vi "Get HW type.vi"(7 "Comm":T1, 8 "error in (no error)":errorcluster) -> (0 "error out":errorcluster, 3 "hwDefaultSetting":T2)   [LabVIEW 2016]
uses:
  Controls/hwDefaultSetting.ctl
  Controls/hwSettings command.ctl
  <vilib>/Utility/config.llb/Read Key (String).vi
  <vilib>/Utility/config.llb/Read Key (U32).vi
  <vilib>/Utility/config.llb/NI_LVConfig.lvlib
panel:
  # "[hw]\nType=Simulation\nhwNumber=2\nhwName=MX840A-1,MX840A-2\nhwSN=0009E5009B32,0009E5009B33\nhwCHNumber=8,8"
  # "I:\\0. iAmleoCHO\\0.09 Projects_ZCJX\\2017\\3. 6Y11S_ZMS_液流台&热气台数据采集\\ZcDAQ\\E\\LabviewPrj\\曹队\\ZcDAQprj\\Builds\\Configuration\n\nI:\\0. iAmleoCHO\\0.09 Projects_ZCJX\\2017\\3. 6Y11S_ZMS_液流台&热气台数据采集\\ZcDAQ\\E\\LabviewPrj\\曹队\\ZcDAQprj\\Builds\\Configuration\\hwtype.ini"
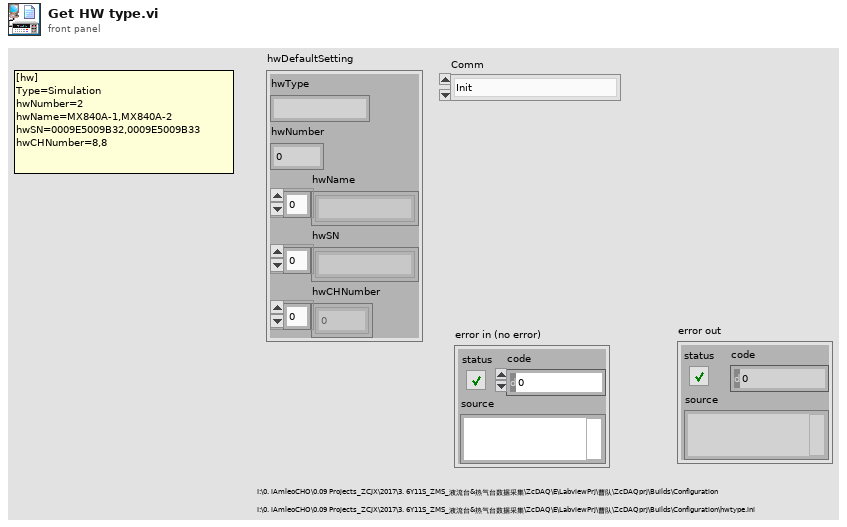
[diagram p1: front panel]
types:
  T1 = typedef "hwSettings command.ctl" = enum16{"Init", "Read", "Clear"}
  T2 = typedef "hwDefaultSetting.ctl" = cluster{"hwType":string, "hwNumber":u32, "hwName":string[], "hwSN":string[], "hwCHNumber":u32[]}
  T3 = cluster{"TREE PNG":path, "User Guide":path, "DefaultSave":path, "BuildPath":path, "Image":path, "Modules":path, "Configuration":path, "License":path, "SplitFiles":path, "System.ini":path}
  T4 = typedef "NI_LVConfig.lvlib/Config Data RefNum.ctl" = refnum<k1>
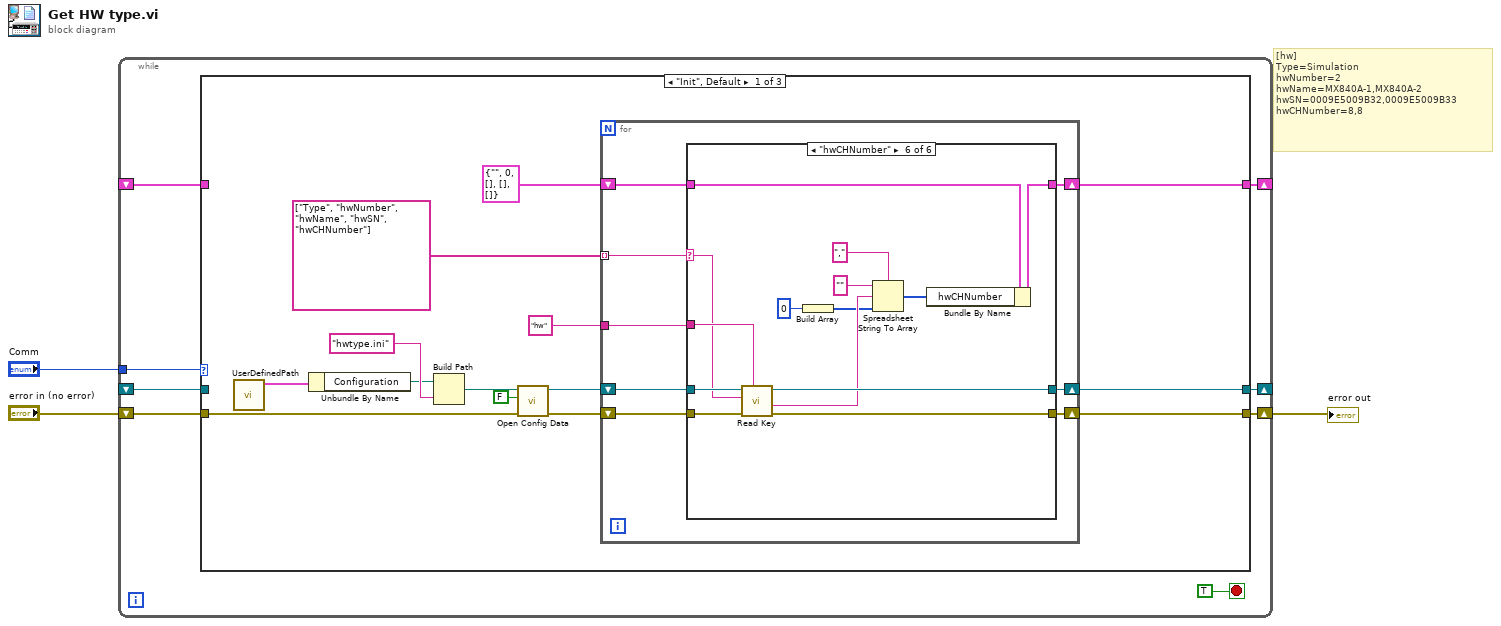
[diagram p0: block diagram]
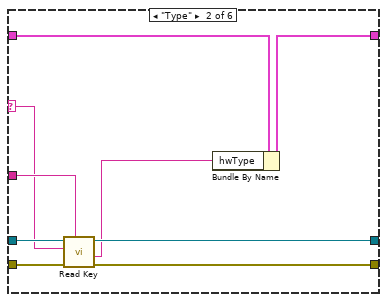
[diagram p3: hidden frame]
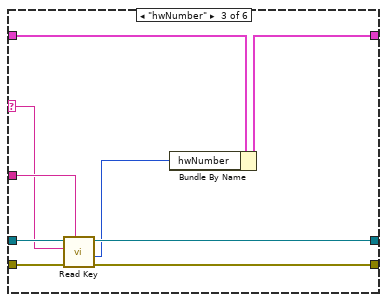
[diagram p4: hidden frame]
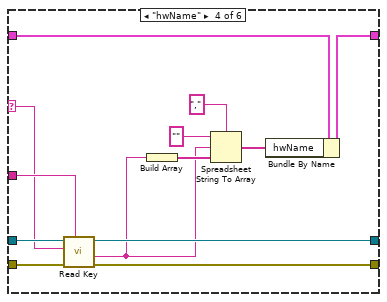
[diagram p5: hidden frame]
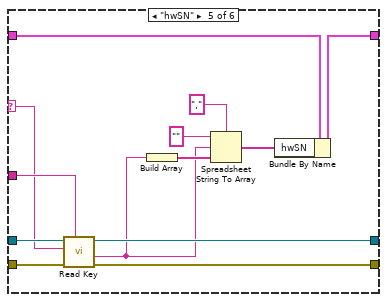
[diagram p6: hidden frame]
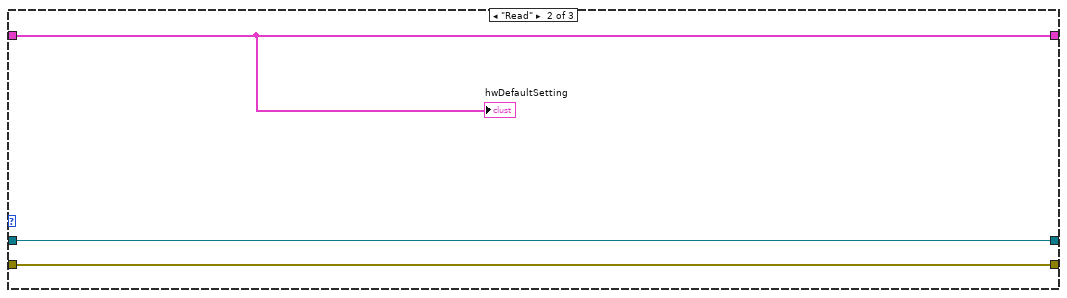
[diagram p7: hidden frame]
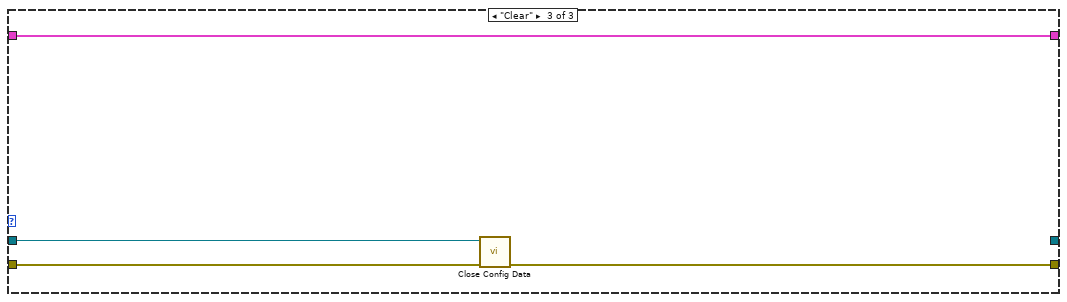
[diagram p8: hidden frame]
diagram:
  # "[hw]\nType=Simulation\nhwNumber=2\nhwName=MX840A-1,MX840A-2\nhwSN=0009E5009B32,0009E5009B33\nhwCHNumber=8,8"
  n1 = while {
    tunnel: "Comm" -> [w10]
    shift-right: [w9] -> _
    shift-left: _ -> [w7]
    shift-right: [w8] -> _
    shift-left: _ -> [w6]
    shift-right: [w4] -> w1
    shift-left: "error in (no error)" -> [w5]
    stop <- TRUE stop-if-true
    n2 = case shown="\"Init\", Default" w10 {
      tunnel: [w15 w97 w101] -> w9
      tunnel: [w14 w96 _] -> w8
      tunnel: w7 -> [_ w97 w101]
      tunnel: w6 -> [_ w96 w100]
      tunnel: w5 -> [w12 w95 w99]
      tunnel: [w13 w95 w98] -> w4
      frame "Init", Default {
        n3 = call "UserDefinedPath.vi"() -> ("UserDefinedPath"=w21:T3)  [unwired: 11 in]
        n4 = Unbundle By Name(w21) -> ("Configuration"=w22:path)
        n5 = Build Path(base path=w22, name or relative path="hwtype.ini") -> (appended path=w24:path)
        n6 = call <vilib>:"Open Config Data.vi"("error in (no error)"=w12, "create file if necessary (T)"=FALSE, "configuration file path"=w24) -> ("error out"=w19:errorcluster, "refnum"=w20:T4)  [unwired: 6 in, 1 out]
        n7 = for {
          shift-right: [w31] -> w14
          shift-left: w20 -> [w33]
          shift-right: [w30] -> w13
          shift-left: w19 -> [w32]
          tunnel: "hw" ("section") -> [w29]
          tunnel: string[] ["Type", "hwNumber", "hwName", "hwSN", "hwCHNumber"] -> [w26] mode=indexing
          shift-right: [w27] -> w15
          shift-left: T2 {"hwType"="", "hwNumber"=0, "hwName"=[], "hwSN"=[], "hwCHNumber"=[]} ("hwDefaultSetting") -> [w28]
          n8 = case shown="\"hwCHNumber\"" w26 {
            selector: w26 -> [_ w38 w47 w60 w73 w87]
            tunnel: w33 -> [w35 w45 w54 w67 w80 w94]
            tunnel: w32 -> [w34 w44 w53 w66 w79 w93]
            tunnel: [w35 w43 w52 w65 w78 w92] -> w31
            tunnel: [w34 w42 w51 w64 w77 w91] -> w30
            tunnel: w29 -> [_ w41 w50 w63 w76 w90]
            tunnel: w28 -> [w36 w40 w49 w62 w75 w89]
            tunnel: [w36 w39 w48 w61 w74 w88] -> w27
            frame Default {
            }
            frame "Type" {
              n9 = call-poly <vilib>:"Read Key.vi"("section"=w41, "error in (no error)"=w44, "key"=w38, "refnum"=w45) -> ("error out"=w42:errorcluster, "value"=w37:string, "refnum out"=w43:T4)  [unwired: 4 in, 1 out]
              n10 = Bundle By Name(cluster=w40, "hwType"=w37) -> (w39:T2)
            }
            frame "hwNumber" {
              n11 = call-poly <vilib>:"Read Key.vi"("section"=w50, "error in (no error)"=w53, "key"=w47, "refnum"=w54) -> ("error out"=w51:errorcluster, "value"=w46:u32, "refnum out"=w52:T4)  [unwired: 4 in, 1 out]
              n12 = Bundle By Name(cluster=w49, "hwNumber"=w46) -> (w48:T2)
            }
            frame "hwName" {
              n13 = call-poly <vilib>:"Read Key.vi"("section"=w63, "error in (no error)"=w66, "key"=w60, "refnum"=w67) -> ("error out"=w64:errorcluster, "value"=w56:string, "refnum out"=w65:T4)  [unwired: 4 in, 1 out]
              n14 = Build Array(w56) -> (w58:string[])
              n15 = Spreadsheet String To Array(delimiter (Tab)=",", format string="", spreadsheet string=w56, array type (2D Dbl)=w58) -> (array=w55:string[])
              n16 = Bundle By Name(cluster=w62, "hwName"=w55) -> (w61:T2)
            }
            frame "hwSN" {
              n17 = call-poly <vilib>:"Read Key.vi"("section"=w76, "error in (no error)"=w79, "key"=w73, "refnum"=w80) -> ("error out"=w77:errorcluster, "value"=w69:string, "refnum out"=w78:T4)  [unwired: 4 in, 1 out]
              n18 = Build Array(w69) -> (w71:string[])
              n19 = Spreadsheet String To Array(delimiter (Tab)=",", format string="", spreadsheet string=w69, array type (2D Dbl)=w71) -> (array=w68:string[])
              n20 = Bundle By Name(cluster=w75, "hwSN"=w68) -> (w74:T2)
            }
            frame "hwCHNumber" {
              n21 = call-poly <vilib>:"Read Key.vi"("section"=w90, "error in (no error)"=w93, "key"=w87, "refnum"=w94) -> ("error out"=w91:errorcluster, "value"=w84:string, "refnum out"=w92:T4)  [unwired: 4 in, 1 out]
              n22 = Build Array(u32 0 ("Numeric")) -> (w83:u32[])
              n23 = Spreadsheet String To Array(delimiter (Tab)=",", format string="", spreadsheet string=w84, array type (2D Dbl)=w83) -> (array=w81:u32[])
              n24 = Bundle By Name(cluster=w89, "hwCHNumber"=w81) -> (w88:T2)
            }
          }
        }
      }
      frame "Read" {
        "hwDefaultSetting" <- w97
      }
      frame "Clear" {
        n25 = call <vilib>:"Close Config Data.vi"("error in (no error)"=w99, "refnum"=w100) -> ("error out"=w98:errorcluster)  [unwired: 8 in, 1 out]
      }
    }
  }
  "error out" <- w1
